vi "Config Curve Header.vi"(0 "VISA resource name":refnum<visa-resource-name>, 1 "Curve Data Format (0: Ohms/K)":u16(ring) items=["Ohms/K", "Log Ohms/K"], 2 "Temp Coefficient (0: Negative)":u16(ring) items=["Negative", "Positive"], 5 "Curve (1)":dbl=1.0 min=1.0 max=20.0 step=1.0, 7 "Curve Name (\"\")":string, 9 "Curve Serial Number (\"\")":string, 11 "error in (no error)":errorcluster, 12 "Limit Value (0.000)":dbl min=0.0 max=1500.0 step=0.001 format="%.3f") -> (4 "VISA resource name out":refnum<visa-resource-name>, 15 "error out":errorcluster)   [LabVIEW 2019, in "Lake Shore Cryotronics 370.lvlib"]
doc: "This VI Configures a user curve header."
uses:
  Lake Shore Cryotronics 370.lvlib
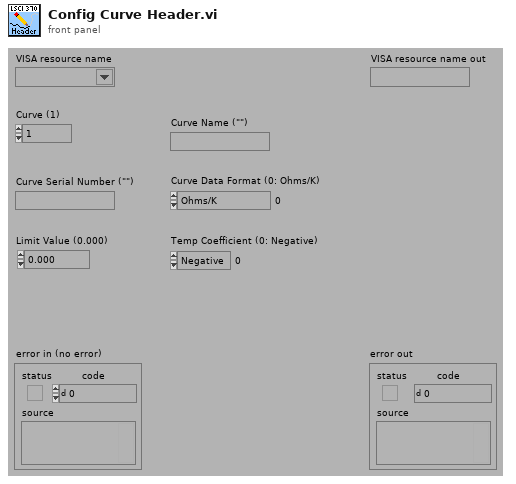
[diagram p1: front panel]
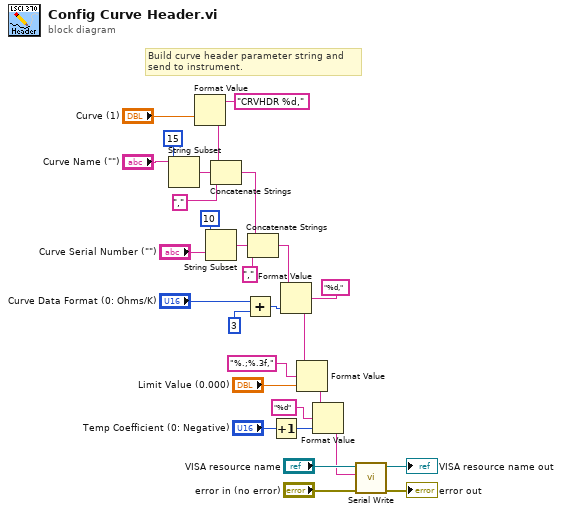
[diagram p0: block diagram]
diagram:
  # "Build curve header parameter string and\nsend to instrument."
  n1 = String Subset(string="Curve Name (\"\")", length (rest)=15) -> (substring=w24:string)  [unwired: 1 in]
  n2 = Format Value(format string="CRVHDR %d,", value (0)="Curve (1)") -> (output string=w25:string)  [unwired: 1 in]
  n3 = String Subset(string="Curve Serial Number (\"\")", length (rest)=10) -> (substring=w28:string)  [unwired: 1 in]
  n4 = Concatenate Strings(w25, w24, ",") -> (w29:string)
  n5 = Add(x="Curve Data Format (0: Ohms/K)", y=3) -> (x+y=w4:i32)
  n6 = Concatenate Strings(w29, w28, ",") -> (w17:string)
  n7 = Increment(x="Temp Coefficient (0: Negative)") -> (x+1=w15:u16)
  n8 = Format Value(string ("")=w17, format string="%d,", value (0)=w4) -> (output string=w1:string)
  n9 = Format Value(string ("")=w1, format string="%.;%.3f,", value (0)="Limit Value (0.000)") -> (output string=w13:string)
  n10 = Format Value(string ("")=w13, format string="%d", value (0)=w15) -> (output string=w5:string)
  n11 = call "Serial Write.vi"("error in (no error)"="error in (no error)", "Write Buffer (\"\")"=w5, "VISA resource name"="VISA resource name") -> ("error out"=→"error out":errorcluster, "VISA resource name out"=→"VISA resource name out":refnum<visa-resource-name>)  [unwired: 6 in, 1 out]
